vi "wuserver.vi"() -> ()   [LabVIEW 2014]
uses:
  <vilib>/addons/zeromq/socket_type.ctl
  <userlib>/_OpenG.lib/numeric/numeric.llb/Random Number Within Range - DBL__ogtk.vi
  <vilib>/addons/zeromq/zmq_context.lvclass
  <vilib>/addons/zeromq/zeromq.lvlib
  <vilib>/addons/zeromq/zmq_socket.lvclass
panel:
  out "relhumidity":string
  out "temperature":string
  out "zipcode":string
  in  "stop":bool
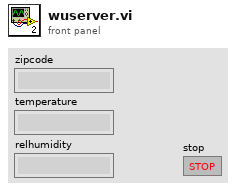
[diagram p1: front panel]
types:
  T1 = typedef "zeromq.lvlib/socket_type.ctl" = enum8{"ZMQ_PAIR", "ZMQ_PUB", "ZMQ_SUB", "ZMQ_REQ", "ZMQ_REP", "ZMQ_DEALER", "ZMQ_ROUTER", "ZMQ_PULL", "ZMQ_PUSH", "ZMQ_XPUB", "ZMQ_XSUB"}
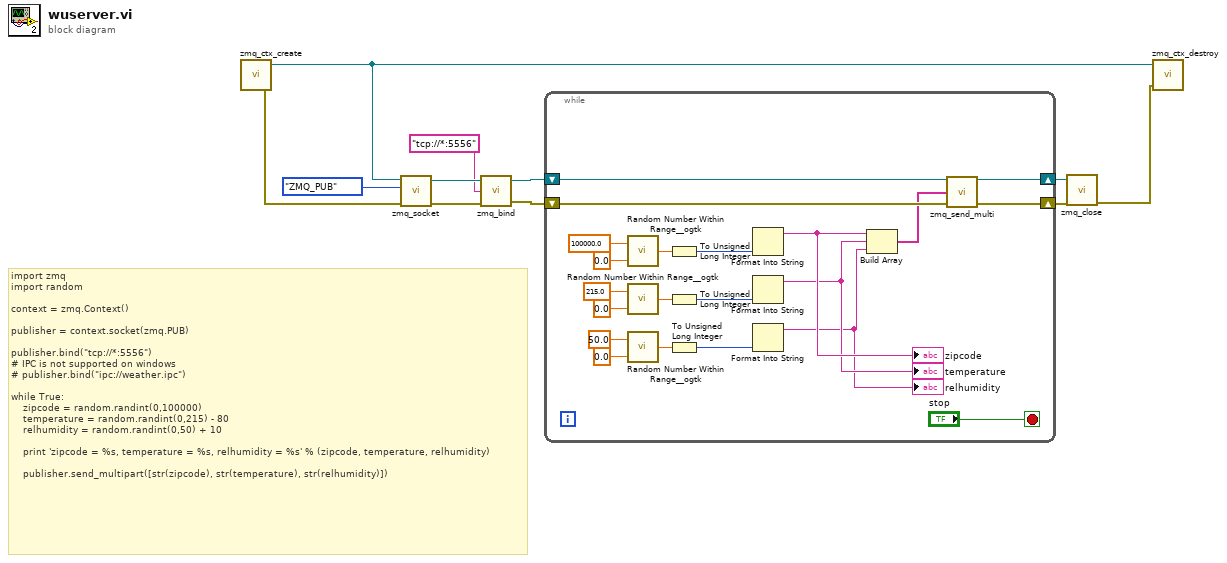
[diagram p0: block diagram]
diagram:
  # "import zmq\nimport random\n\ncontext = zmq.Context()\n\npublisher = context.socket(zmq.PUB)\n\npublisher.bind(\"tcp://*:5556\")\n# IPC is not supported on windows\n# publisher.bind(\"ipc://weather.ipc\")\n\nwhile True:\n    zipcode = random.randint(0,100000)\n    temperature = random.randint(0,215) - 80\n    relhumidity = random.randint(0,50) + 10\n\n    print 'zipcode = %s, temperature = %s, relhumidity = %s' % (zipcode, temperature, relhumidity)\n\n    publisher.send_multipart([str(zipcode), str(temperature), str(relhumidity)])"
  n1 = call <vilib>:"zmq_ctx_create.vi"() -> ("error out"=w10:errorcluster, "context out"=w9:refnum<class "zmq_context.lvclass">)  [unwired: 4 in]
  n2 = call <vilib>:"zmq_socket.vi"("error in"=w10, "socket type"=socket_type."ZMQ_PUB", "context in"=w9) -> ("error out"=w7:errorcluster, "socket out"=w8:refnum<class "zmq_socket.lvclass">)  [unwired: 2 in, 1 out]
  n3 = call <vilib>:"zmq_bind.vi"("error in"=w7, "endpoint"="tcp://*:5556", "socket in"=w8) -> ("error out"=w4:errorcluster, "socket out"=w5:refnum<class "zmq_socket.lvclass">)  [unwired: 1 in]
  n4 = while {
    shift-right: [w30] -> w3
    shift-left: w5 -> [w32]
    shift-right: [w29] -> w2
    shift-left: w4 -> [w31]
    stop <- "stop" stop-if-true
    n5 = call-poly <userlib>:"Random Number Within Range__ogtk.vi"("High"=100000.0, "Low"=0.0) -> ("Random Number"=w21:dbl)  [unwired: 3 in]
    n6 = call-poly <userlib>:"Random Number Within Range__ogtk.vi"("High"=215.0, "Low"=0.0) -> ("Random Number"=w18:dbl)  [unwired: 3 in]
    n7 = call-poly <userlib>:"Random Number Within Range__ogtk.vi"("High"=50.0, "Low"=0.0) -> ("Random Number"=w19:dbl)  [unwired: 3 in]
    n8 = To Unsigned Long Integer(number=w21) -> (unsigned 32bit integer=w20:u32)
    n9 = To Unsigned Long Integer(number=w18) -> (unsigned 32bit integer=w13:u32)
    n10 = To Unsigned Long Integer(number=w19) -> (unsigned 32bit integer=w12:u32)
    n11 = Format Into String(w20) -> (resulting string=w17:string)  [unwired: 3 in, 1 out]
    "zipcode" <- w17
    n12 = Format Into String(w13) -> (resulting string=w15:string)  [unwired: 3 in, 1 out]
    "temperature" <- w15
    n13 = Format Into String(w12) -> (resulting string=w14:string)  [unwired: 3 in, 1 out]
    "relhumidity" <- w14
    n14 = Build Array(w17, w15, w14) -> (w16:string[])
    n15 = call <vilib>:"zmq_send_multi.vi"("error in"=w31, "parts"=w16, "socket in"=w32) -> ("error out"=w29:errorcluster, "socket out"=w30:refnum<class "zmq_socket.lvclass">)  [unwired: 1 in]
  }
  n16 = call <vilib>:"zmq_close.vi"("error in"=w2, "socket"=w3) -> ("error out"=w1:errorcluster)  [unwired: 3 in]
  n17 = call <vilib>:"zmq_ctx_destroy.vi"("error in"=w1, "context in"=w9) -> ()  [unwired: 3 in, 1 out]
